vi "dfd_FXP Add.vi"   [LabVIEW 2017, in "NI_DigFilter_FXP.lvlib"]
uses:
  <vilib>/addons/Digital Filter Design/NI_DigFilter_FXP.lvlib
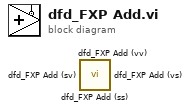
[diagram p0: block diagram]
diagram:
  n1 = call <vilib>:"dfd_FXP Add (ss).vi"() -> ()  [unwired: 6 in, 3 out]
  n2 = call <vilib>:"dfd_FXP Add (vv).vi"() -> ()  [unwired: 6 in, 3 out]
  n3 = call <vilib>:"dfd_FXP Add (sv).vi"() -> ()  [unwired: 6 in, 3 out]
  n4 = call <vilib>:"dfd_FXP Add (vs).vi"() -> ()  [unwired: 6 in, 3 out]
